vi "FindFocus.vi"(8 "error in (no error)":errorcluster, 11 "Transport":refnum<class "Transport.lvclass">) -> (0 "error out":errorcluster, 3 "Transport.lvclass":refnum<class "Transport.lvclass">)   [LabVIEW 2019, in "Transport.lvclass"]
uses:
  <userlib>/LevyLab/Transport/Transport/Transport.lvclass
  <userlib>/LevyLab/Instrument Framework/Instrument Types/Cryostat/Instrument.Cryostat.lvclass
  <userlib>/LevyLab/Transport/Control Experiment/Control Experiment.lvclass
  <userlib>/LevyLab/Krohn Hite 7008/Instrument.KH7008.lvclass
  <userlib>/LevyLab/Lockin-Multichannel/Instrument.Lockin/Instrument.Lockin.lvclass
  <userlib>/LevyLab/Transport/Control Experiment/Typedefs/Instruments--cluster.ctl
  <userlib>/LevyLab/Instrument Framework/Instrument Types/VSource/Instrument.VSource.lvclass
  <userlib>/LevyLab/Instrument Framework/Instrument Types/VNA/Instrument.VNA.lvclass
  <userlib>/LevyLab/Instrument Framework/Instrument Types/Strain/Instrument.Strain.lvclass
  <userlib>/LevyLab/Instrument Framework/Instrument Types/CBridge/Instrument.CBridge.lvclass
  <userlib>/LevyLab/Instrument Framework/Instrument Types/Delay Line/Instrument.DelayLine.lvclass
  <userlib>/LevyLab/Lockin-Multichannel/Instrument.Lockin/Typedefs/Results Type--Enum.ctl
panel:
  in  "set \"Vsg\" to initial value?":bool
  in  "Tab Control":enum32{"LockIn Control", "Data", "Other"}(tab)
  out "elapsed time (s)":u32=1660
  in  "Input":i32[](array[numeric])=[21]
  in  "End (um)":dbl=10.0 format="%#_3p"
  in  "Start (um)":dbl format="%#_3p"
  in  "Step (um)":dbl=0.1 format="%#_3p"
  in  "Experiment Comments":string
  in  "Experiment Folder":string="Focus Optimization xxxxxxxx"
  out "T (mK)":dbl=0.001
  in  "wait after setting Control (ms)":u32=2000
  in  "Initial wait (ms)":u32=1000
  in  "Sweep":enum16{"Vsg", "Vbg", "Z-height", ""}(ring)=enum."Z-height"
  in  "cycles (1,2,...)":i32=1 min=1 step=1
  in  "phase":dbl
  out "Field (T)":dbl=-0.0003 format="%#_13g"
  in  "function (ramp)":enum16{"Ramp", "Triangle", "Sine"}(ring)
  out "time b/w points (ms)":u32=2066
  in  "stop":bool
  out "Mean vs. Parameter":cluster{dbl[], dbl[]}[](graph)
  out "X Lockins":cluster{dbl[], dbl[]}[](graph)
  out "Y Lockins":cluster{dbl[], dbl[]}[](graph)
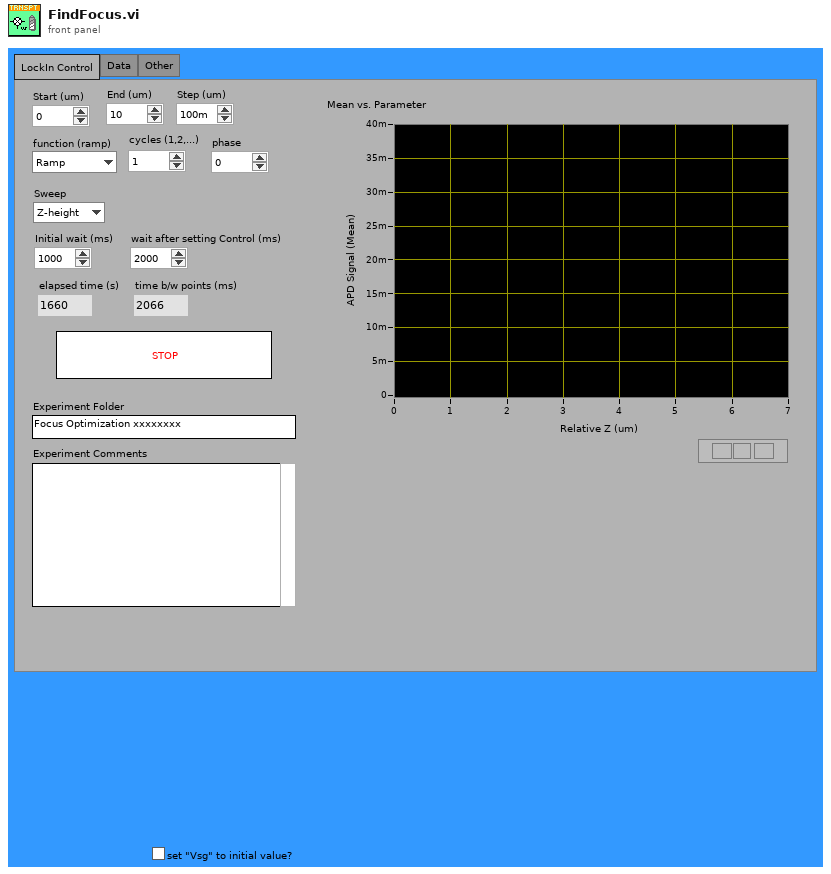
[diagram p1: front panel]
types:
  T1 = enum32{"Invalid", "Standard", "Closed", "Hidden", "Minimized", "Maximized"}
  T2 = enum32{"invalid app kind", "Development System", "Run Time System", "Student Edition", "Embedded LabVIEW", "Evaluation", "Custom"}
  T3 = typedef "Instrument.Lockin.lvclass/Results Type--Enum.ctl" = enum16{"X", "Y", "R", "Theta", "Mean"}
  T4 = typedef "Control Experiment.lvclass/Instruments--cluster.ctl" = cluster{"KH7008":refnum<class "Instrument.KH7008.lvclass">[], "Lockin":refnum<class "Instrument.Lockin.lvclass">, "Temperature":refnum<class "Instrument.Cryostat.lvclass">, "Magnet":refnum<class "Instrument.Cryostat.lvclass">, "Rotator":refnum<class "Instrument.Cryostat.lvclass">, "Level":refnum<class "Instrument.Cryostat.lvclass">, "Capacitance Bridge":refnum<class "Instrument.CBridge.lvclass">, "Delay Line":refnum<class "Instrument.DelayLine.lvclass">, "Strain Cell":refnum<class "Instrument.Strain.lvclass">, "VNA":refnum<class "Instrument.VNA.lvclass">, "Voltage Source":refnum<class "Instrument.VSource.lvclass">}
  T5 = cluster{"Core":cluster{"Current VI Reference":refnum<vi>, "Close Panel on Exit?":bool}, "Transport":refnum<class "Transport.lvclass">, "C.E.":refnum<class "Control Experiment.lvclass">, "Instruments":T4, "Sweep Values":dbl[], "Results (Dictionary)":cluster{"key":string, "value":dbl}[], "size":i32, "index":i32, "ms [0]":u32, "ms [i]":u32, "Execution:State":enum32{"Bad", "Idle", "Run top level", "Running"}}
  T6 = enum32{"Bad", "Idle", "Run top level", "Running"}
  T7 = cluster{"Current VI Reference":refnum<vi>, "Close Panel on Exit?":bool}
  T8 = cluster{"I-":i32, "I+":i32, "V1-":i32, "V1+":i32, "I2-":i32, "I2+":i32, "V2-":i32, "V2+":i32}
  T9 = typedef "Instrument.DAQ.lvclass/AO.Channel--Cluster--Array.ctl" = T10[]
  T10 = typedef "Instrument.DAQ.lvclass/AO.Channel--Cluster.ctl" = cluster{"Enable?":bool, "Channel":i32, "Amplitude":dbl, "Offset":dbl, "Frequency":dbl, "Phase":dbl, "Function":T11, "Sweeping?":bool}
  T11 = typedef "Instrument.DAQ.lvclass/AO.Channel.Function--Enum.ctl" = enum16{"Sine", "Triangle", "Square"}
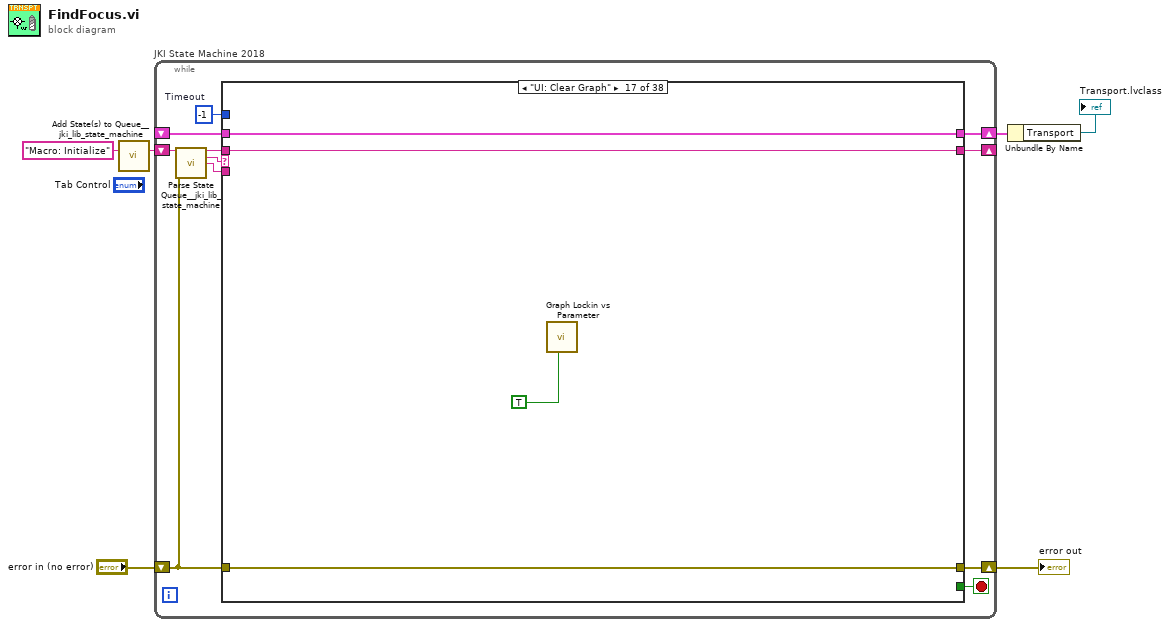
[diagram p0: block diagram]
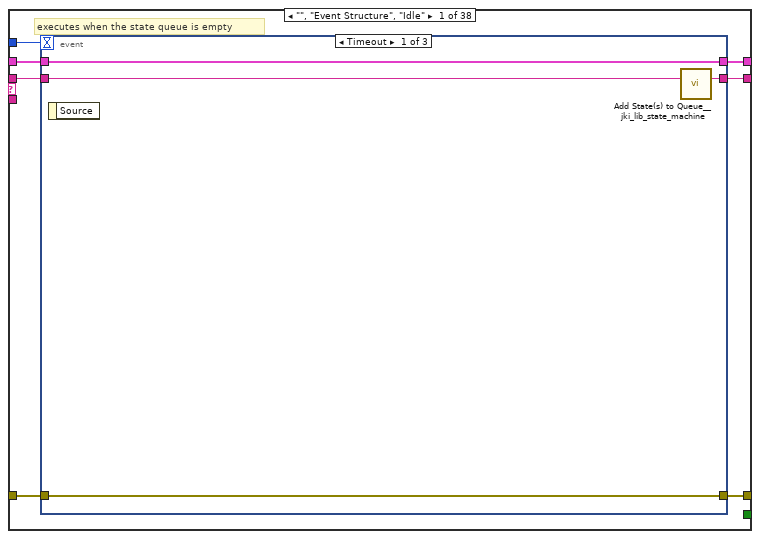
[diagram p2: hidden frame]
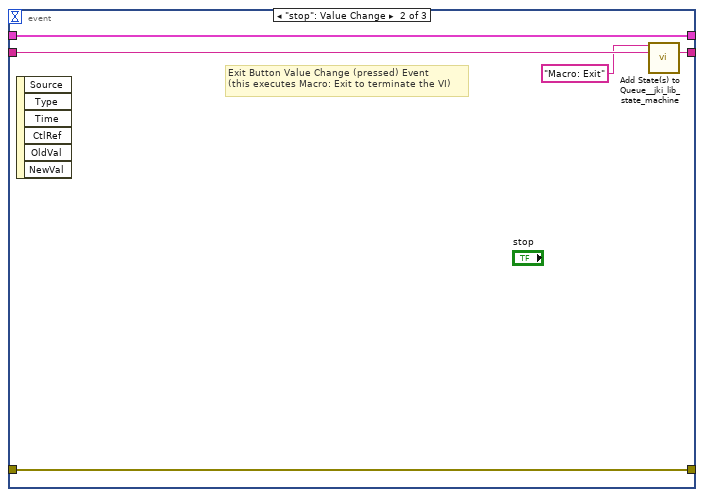
[diagram p3: hidden frame]
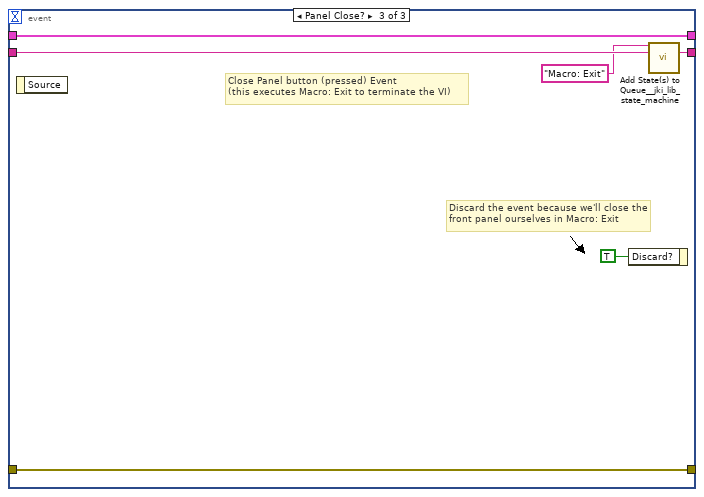
[diagram p4: hidden frame]
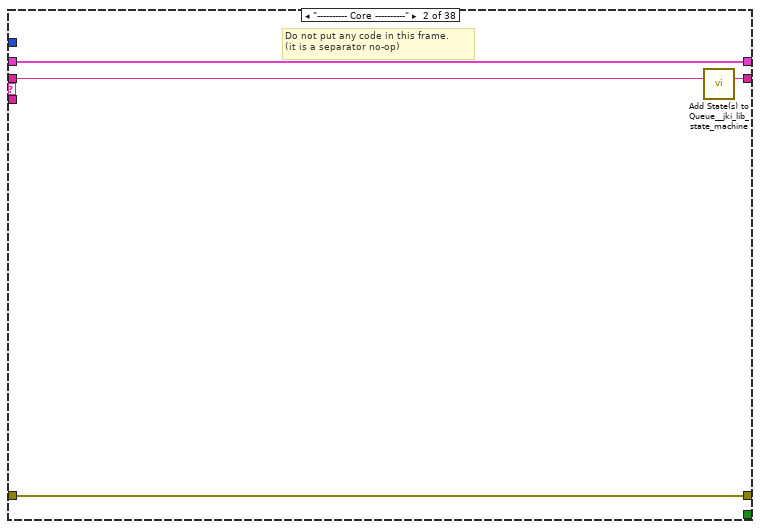
[diagram p5: hidden frame]
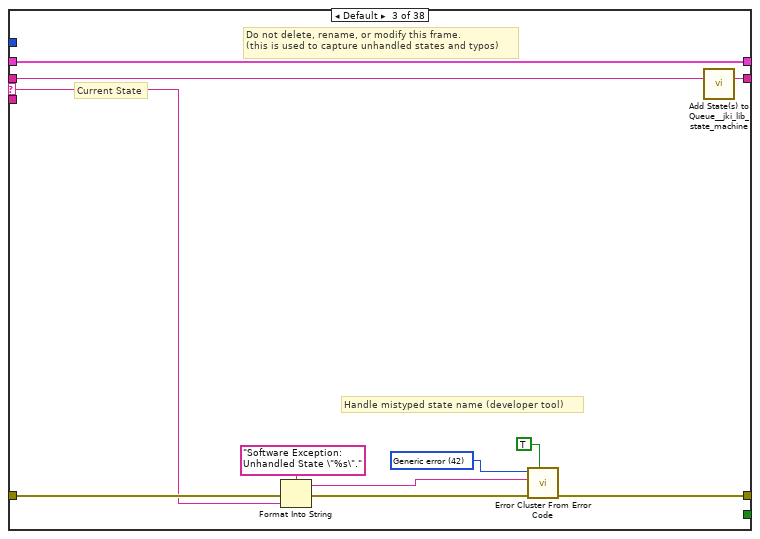
[diagram p6: hidden frame]
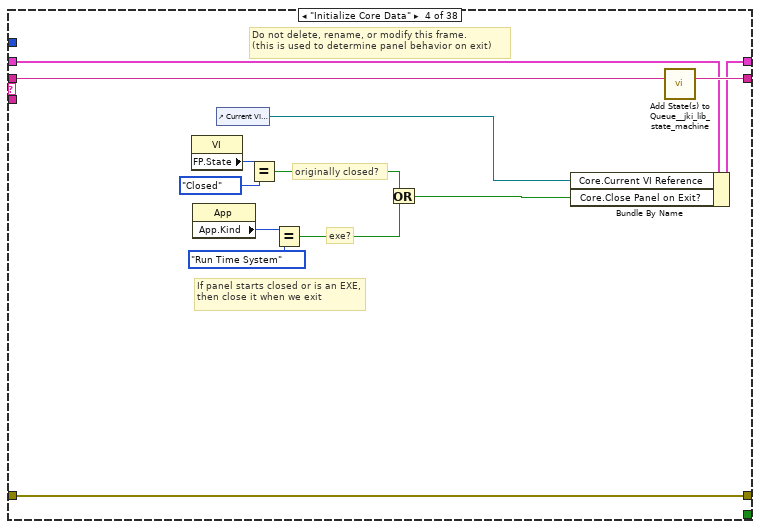
[diagram p7: hidden frame]
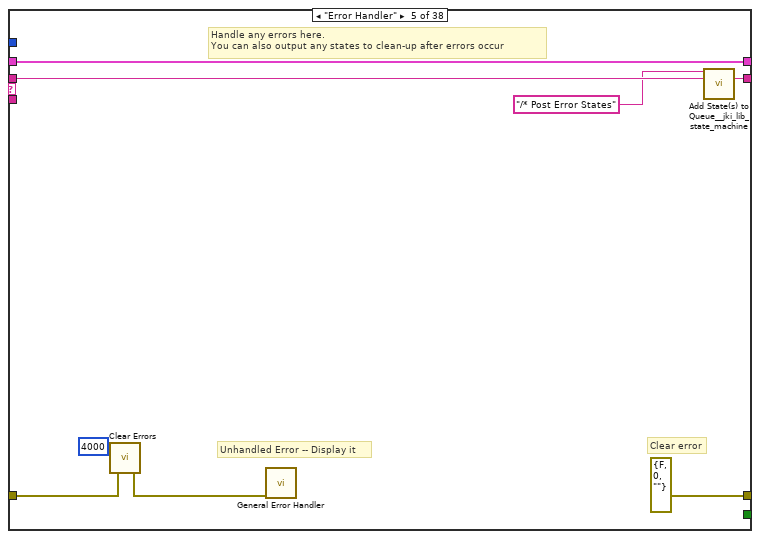
[diagram p8: hidden frame]
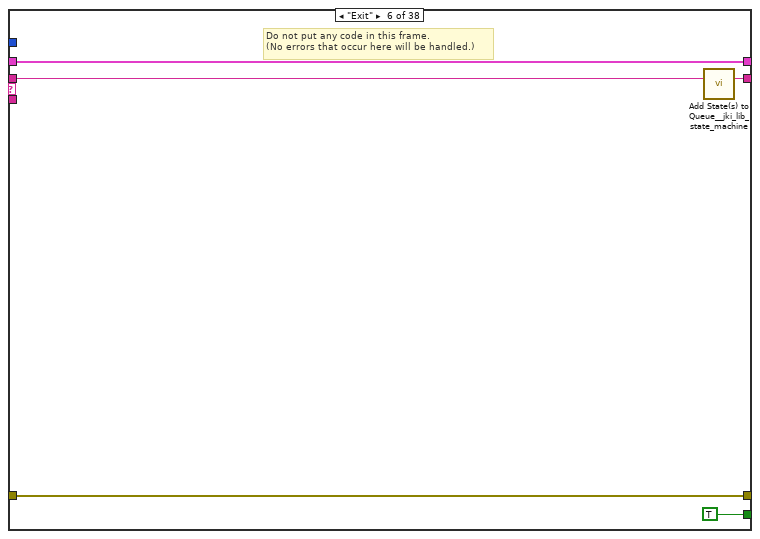
[diagram p9: hidden frame]
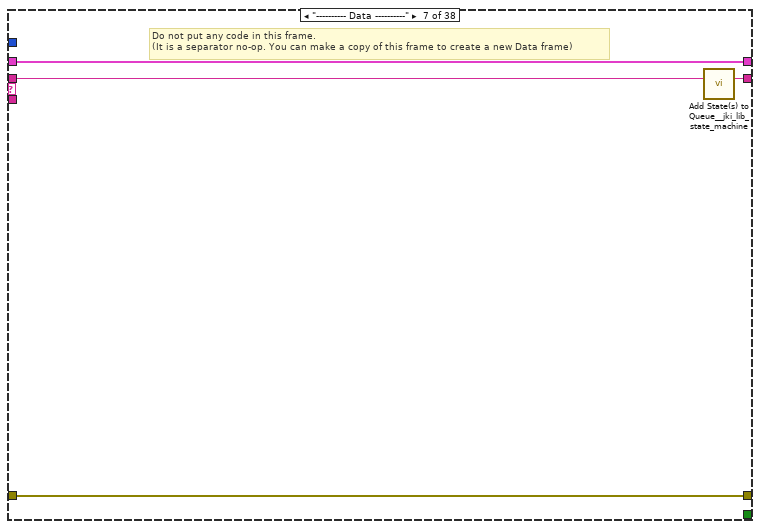
[diagram p10: hidden frame]
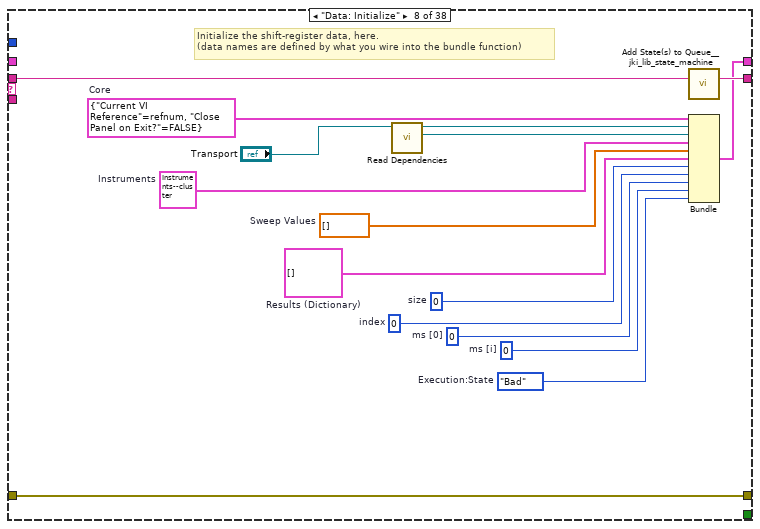
[diagram p11: hidden frame]
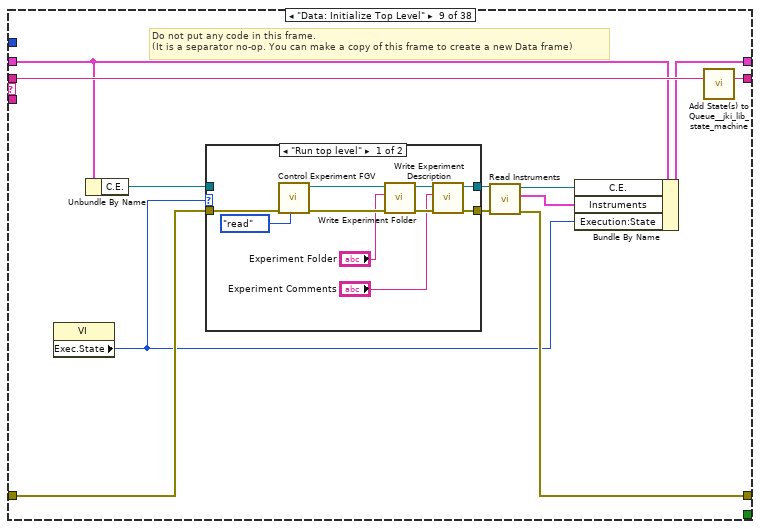
[diagram p12: hidden frame]
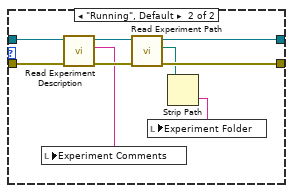
[diagram p13: hidden frame]
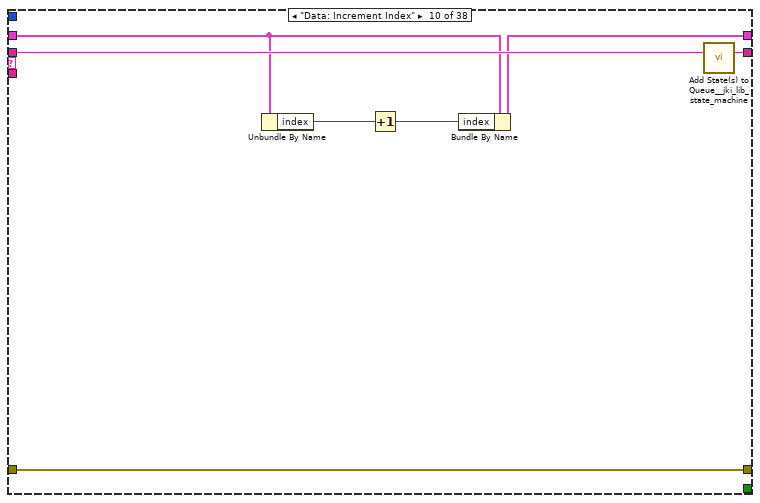
[diagram p14: hidden frame]
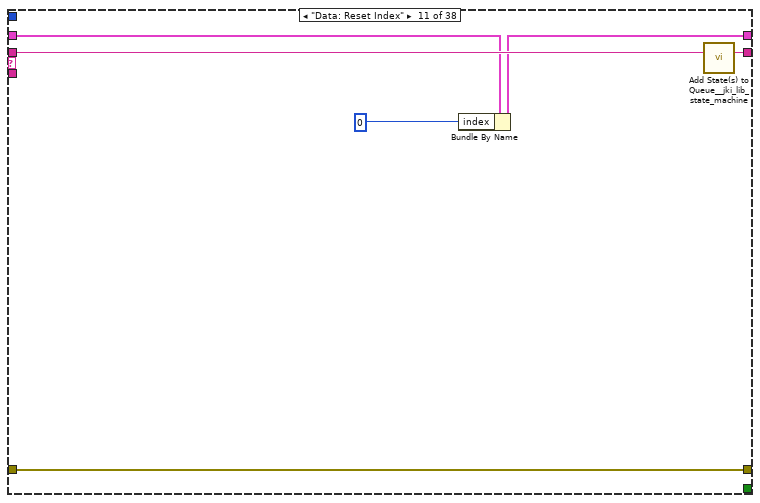
[diagram p15: hidden frame]
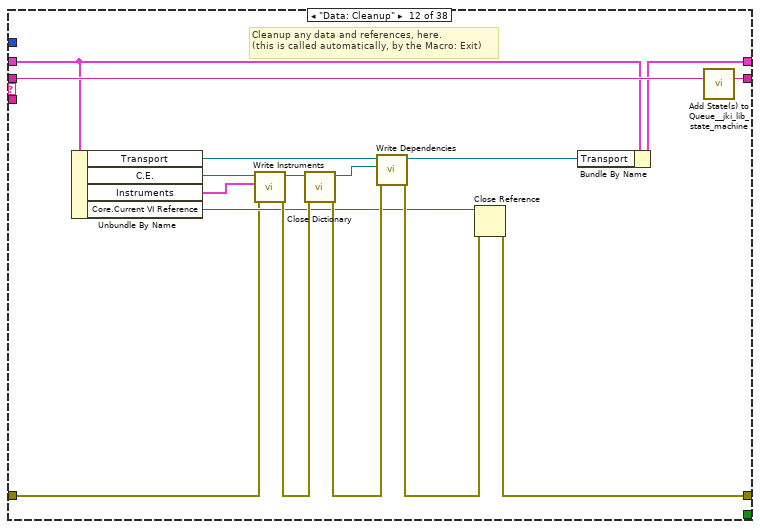
[diagram p16: hidden frame]
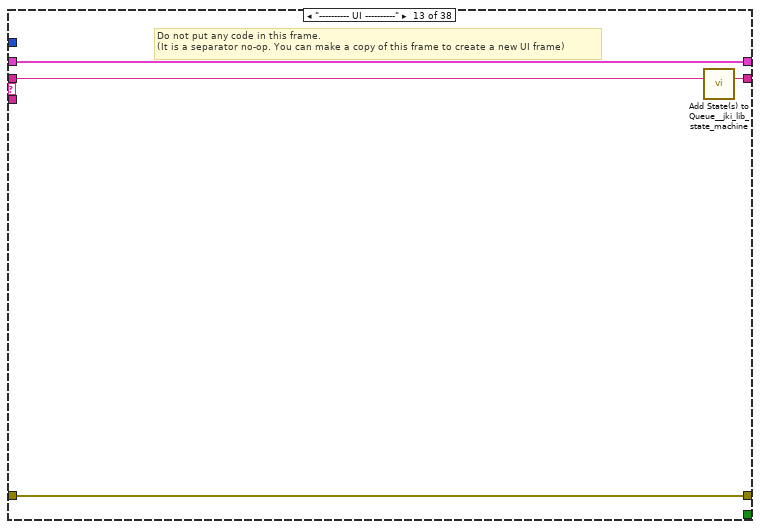
[diagram p17: hidden frame]
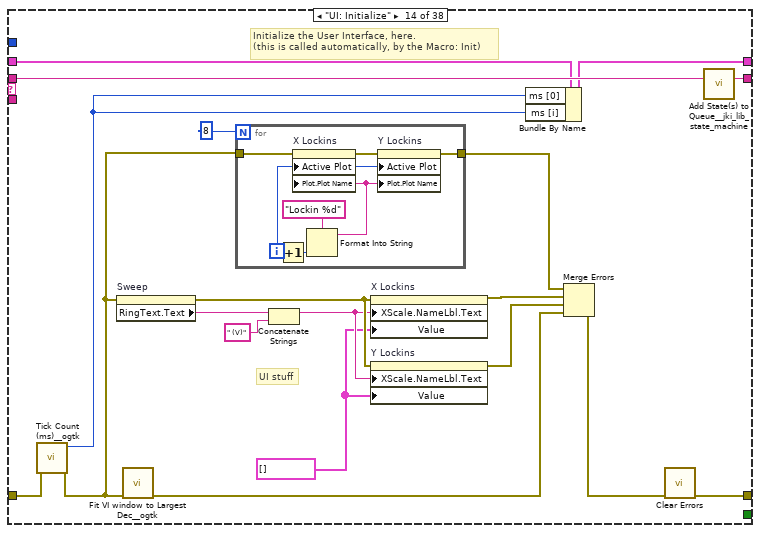
[diagram p18: hidden frame]
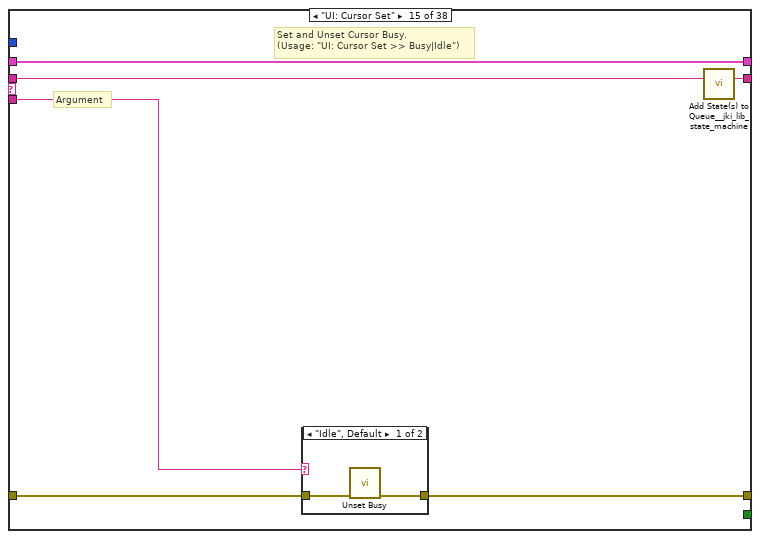
[diagram p19: hidden frame]
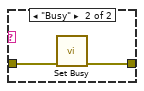
[diagram p20: hidden frame]
diagram:
  n1 = call <vilib>:"Add State(s) to Queue__jki_lib_state_machine.vi"("State(s) in (\"\")"="Macro: Initialize") -> ("States Out"=w6:string)  [unwired: 14 in]
  n2 = while "JKI State Machine 2018" {
    shift-right: [w10] -> w4
    shift-left: _ -> [w9]
    shift-right: [w13] -> w2
    shift-left: "error in (no error)" -> [w7]
    shift-right: [w12] -> _
    shift-left: w6 -> [w14]
    stop <- w11 stop-if-true
    w8 = -1  # Timeout
    n3 = call <vilib>:"Parse State Queue__jki_lib_state_machine.vi"("State Queue"=w14, "Error In (no error)"=w7) -> ("Remaining States"=w16:string, "Current State"=w17:string, "Arguments"=w15:string)  [unwired: 11 in]
    n4 = case shown="\"UI: Clear Graph\"" w17 {
      selector: w17 -> [_ _ w44 _ _ _ _ _ _ _ _ _ _ _ _ _ _ _ _ _ _ _ _ _ _ _ _ _ _ _ _ _ _ _ _ _ _ _]
      tunnel: w16 -> [w24 w43 w48 w67 w75 w80 w84 w100 w112 w138 w144 w160 w164 w183 w196 w216 w219 w233 w240 w309 w314 w336 w346 w350 w378 w390 w397 w411 w466 w479 w492 w505 w523 w555 w566 w570 w574 w583]
      tunnel: w15 -> [_ _ _ _ _ _ _ _ _ _ _ _ _ _ w191 _ _ _ w234 _ _ _ _ _ _ _ _ _ _ _ _ _ _ _ _ _ _ _]
      tunnel: w9 -> [w22 w40 w46 w60 w72 w78 w81 _ w103 w132 w141 w148 w161 w168 w194 w209 w220 w228 w236 w306 w312 w329 w343 w347 w366 w387 w393 w401 w463 w475 w489 w500 w518 w552 w562 w567 w571 w577]
      tunnel: [w21 w41 w50 w64 errorcluster {"status"=FALSE, "code"=0, "source"=""} ("error out") w77 w82 w97 w104 w136 w142 w145 w162 w173 w192 w214 w218 w222 w237 w307 w310 w334 w344 w348 w356 w388 w394 w405 w464 w471 w483 w496 w514 w546 w557 w568 w572 w580] -> w13
      tunnel: w7 -> [w20 w41 w49 w64 w69 w77 w82 w97 w105 w136 w142 w146 w162 w170 w193 w214 w218 w230 w238 w307 w310 w334 w344 w348 w363 w388 w395 w404 w464 w476 w487 w497 w521 w547 w558 w568 w572 w579]
      tunnel: [w23 w42 w47 w66 w74 w79 w83 w99 w111 w137 w143 w159 w163 w182 w195 w215 w219 w232 w239 w308 w313 w335 w345 w349 w377 w389 w396 w410 w465 w478 w491 w504 w522 w554 w565 w569 w573 w582] -> w12
      tunnel: [_ _ _ _ _ TRUE _ _ _ _ _ _ _ _ _ _ _ _ _ _ _ _ _ _ _ _ _ _ _ _ _ _ _ _ _ _ _ _] -> w11
      tunnel: [w19 w40 w46 w65 w72 w78 w81 w98 w102 w135 w140 w147 w161 w167 w194 w209 w220 w227 w236 w306 w312 w329 w343 w347 w369 w387 w393 w402 w463 w474 w488 w499 w519 w553 w563 w567 w571 w576] -> w10
      tunnel: w8 -> [w18 _ _ _ _ _ _ _ _ _ _ _ _ _ _ _ _ _ _ _ _ _ _ _ _ _ _ _ _ _ _ _ _ _ _ _ _ _]
      frame "", "Event Structure", "Idle" {
        # "executes when the state queue is empty"
        n5 = event shown="[0] Timeout" {
          selector: _ -> [_ _ _]
          dyn-events: _ -> [_ _ _]
          timeout: w18 -> [_ _ _]
          tunnel: w24 -> [w28 w33 w39]
          tunnel: [w27 w32 w38] -> w23
          tunnel: w22 -> [w25 w30 w36]
          tunnel: [w26 w31 w37] -> w21
          tunnel: w20 -> [w26 w31 w37]
          tunnel: [w25 w30 w36] -> w19
          event Timeout {
            n6 = event-data() -> ()  [unwired: 1 in, 1 out]
            n7 = call <vilib>:"Add State(s) to Queue__jki_lib_state_machine.vi"("State(s) in (\"\")"=w28) -> ("States Out"=w27:string)  [unwired: 14 in]
          }
          event "stop": Value Change {
            # "Exit Button Value Change (pressed) Event\n(this executes Macro: Exit to terminate the VI)"
            n8 = event-data() -> ()  [unwired: 1 in, 6 out]
            n9 = call <vilib>:"Add State(s) to Queue__jki_lib_state_machine.vi"("State(s) in Front (\"\")"="Macro: Exit", "State(s) in (\"\")"=w33) -> ("States Out"=w32:string)  [unwired: 13 in]
          }
          event Panel Close? {
            # "Discard the event because we'll close the front panel ourselves in Macro: Exit"
            # "Close Panel button (pressed) Event\n(this executes Macro: Exit to terminate the VI)"
            n10 = event-data() -> ()  [unwired: 1 in, 1 out]
            n11 = event-data("Discard?"=TRUE) -> ()  [unwired: 1 in, 1 out]
            n12 = call <vilib>:"Add State(s) to Queue__jki_lib_state_machine.vi"("State(s) in Front (\"\")"="Macro: Exit", "State(s) in (\"\")"=w39) -> ("States Out"=w38:string)  [unwired: 13 in]
          }
        }
      }
      frame "---------- Core ----------" {
        # "Do not put any code in this frame.\n(it is a separator no-op)"
        n13 = call <vilib>:"Add State(s) to Queue__jki_lib_state_machine.vi"("State(s) in (\"\")"=w43) -> ("States Out"=w42:string)  [unwired: 14 in]
      }
      frame Default {
        w53 = 42 items=["No error", "Argument error", "Memory is full", "Out of zone", "End of file", "File already open", "Generic file I/O error", "File not found", "File permission error", "Disk is full", "Duplicate path", "Too many files open", "System feature not enabled", "Resource file not found", "Cannot add resource", "Resource not found", "Image not found", "Image memory error", "Pen does not exist", "Config type invalid", "Config token not found", "Config parse error", "Config memory error", "Bad external code format", "Bad external code offset", "External code not present", "Null window", "Destroy window error", "Null menu", "Print aborted", "Bad print record", "Print driver error", "Windows error during printing", "Memory error during printing", "Print dialog error", "Generic print error", "Invalid device refnum", "Device not found", "Device parameter error", "Device unit error", "Cannot open device", "Device call aborted", "Generic error", "Cancelled by user", "Object ID too low", "Object ID too high", "Object not in heap", "Unknown heap", "Unknown object (invalid DefProc)", "Unknown object (DefProc not in table)", "Message out of range", "Invalid (null) method", "Unknown message", "Manager call not supported", "Bad address", "Network operation in progress", "Network operation timed out", "Connection is busy", "Network attribute not supported", "Network error", "Address in use", "System out of memory", "Connection aborted", "Connection refused", "Not connected", "Already connected", "Connection closed", "Initialization error (interapplication manager)", "Bad occurrence", "Wait on unbound occurrence handler", "Occurrence queue overflow", "Datalog type conflict", "Unused", "Unrecognized type (interapplication manager)", "Memory corrupt", "Failed to make temporary DLL", "Old CIN version", "Drag socket not found", "Failed to load drop-object", "Failed to register OLE object", "Failed to release OLE object", "Format specifier type mismatch", "Unknown format specifier", "Too few format specifiers", "Too many format specifiers", "Scan failed", "Newer CIN version", "Error converting to variant", "Runtime menu error", "Password tampered", "Variant attribute not found", "Incompatible variant data type", "Event data is not available", "Event Store is not present", "Occurrence is not found", "Event Queue is not created", "Event info is not available", "Refnum passed is NULL", "Error retrieving Class GUID", "Error retrieving CoClass GUID", "Error retrieving TypeLib GUID.", "Bad built application magic bytes.", "Specific driver is different from the specific driver associated with the Logical Name.", "There is no session opened to the class driver.", "Max Error", "MAX - Error with config objects", "MAX - Error loading configuration", "MAX - Group not supported"]
        # "Current State"
        # "Do not delete, rename, or modify this frame.\n(this is used to capture unhandled states and typos)"
        # "Handle mistyped state name (developer tool)"
        n14 = Format Into String(format string="Software Exception: Unhandled State \"%s\"." ("message"), error in=w49, w44) -> (resulting string=w52:string, error out=w51:errorcluster)  [unwired: 1 in]
        n15 = call <vilib>:"Error Cluster From Error Code.vi"("show call chain? (False)"=TRUE, "error in (no error)"=w51, "error message (\"\")"=w52, "error code (0)"=w53) -> ("error out"=w50:errorcluster)  [unwired: 5 in]
        n16 = call <vilib>:"Add State(s) to Queue__jki_lib_state_machine.vi"("State(s) in (\"\")"=w48) -> ("States Out"=w47:string)  [unwired: 14 in]
      }
      frame "Initialize Core Data" {
        # "Do not delete, rename, or modify this frame.\n(this is used to determine panel behavior on exit)"
        # "originally closed?"
        # "exe?"
        # "If panel starts closed or is an EXE, then close it when we exit"
        n17 = property class="VI"() -> ("FP.State"=w57:T1)  [unwired: 2 in, 2 out]
        n18 = property class="App"() -> ("App.Kind"=w63:T2)  [unwired: 2 in, 2 out]
        n19 = control-ref of="Current VI Reference"() -> (w58:refnum<vi>)
        n20 = Equal?(x=w57, y=T1."Closed" ("Front Panel Window:State")) -> (x = y?=w55:bool)
        n21 = Equal?(x=w63, y=T2."Run Time System" ("Application:Kind")) -> (x = y?=w61:bool)
        n22 = Or(x=w55, y=w61) -> (x .or. y?=w59:bool)
        n23 = Bundle By Name(cluster=w60, "Core.Current VI Reference"=w58, "Core.Close Panel on Exit?"=w59) -> (w65:T5)
        n24 = call <vilib>:"Add State(s) to Queue__jki_lib_state_machine.vi"("State(s) in (\"\")"=w67) -> ("States Out"=w66:string)  [unwired: 14 in]
      }
      frame "Error Handler" {
        # "Unhandled Error -- Display it"
        # "Handle any errors here.\nYou can also output any states to clean-up after errors occur"
        # "Clear error"
        n25 = call <vilib>:"Clear Errors.vi"("error in (no error)"=w69, "specific error code to clear (0: all)"=4000) -> ("error out"=w68:errorcluster)  [unwired: 4 in, 1 out]
        n26 = call <vilib>:"General Error Handler.vi"("error in (no error)"=w68) -> ()  [unwired: 10 in, 5 out]
        n27 = call <vilib>:"Add State(s) to Queue__jki_lib_state_machine.vi"("State(s) in Front (\"\")"="/* Post Error States", "State(s) in (\"\")"=w75) -> ("States Out"=w74:string)  [unwired: 13 in]
      }
      frame "Exit" {
        # "Do not put any code in this frame.\n(No errors that occur here will be handled.)"
        n28 = call <vilib>:"Add State(s) to Queue__jki_lib_state_machine.vi"("State(s) in (\"\")"=w80) -> ("States Out"=w79:string)  [unwired: 14 in]
      }
      frame "---------- Data ----------" {
        # "Do not put any code in this frame.\n(It is a separator no-op. You can make a copy of this frame to create a new Data frame)"
        n29 = call <vilib>:"Add State(s) to Queue__jki_lib_state_machine.vi"("State(s) in (\"\")"=w84) -> ("States Out"=w83:string)  [unwired: 14 in]
      }
      frame "Data: Initialize" {
        w85 = cluster{"key":string, "value":dbl}[] []  # Results (Dictionary)
        w89 = T6."Bad"  # Execution:State
        w90 = 0  # size
        w91 = u32 0  # ms [i]
        w92 = u32 0  # ms [0]
        w93 = 0  # index
        w94 = dbl[] []  # Sweep Values
        w95 = T4 {"KH7008"=[], "Lockin"=refnum, "Temperature"=refnum, "Magnet"=refnum, "Rotator"=refnum, "Level"=refnum, "Capacitance Bridge"=refnum, "Delay Line"=refnum, "Strain Cell"=refnum, "VNA"=refnum, "Voltage Source"=refnum}  # Instruments
        w96 = T7 {"Current VI Reference"=refnum, "Close Panel on Exit?"=FALSE}  # Core
        # "Initialize the shift-register data, here.\n(data names are defined by what you wire into the bundle function)"
        n30 = call <userlib>:"Read Dependencies.vi"("Transport"="Transport") -> ("C.E."=w87:refnum<class "Control Experiment.lvclass">, "Transport"=w86:refnum<class "Transport.lvclass">)  [unwired: 8 in, 1 out]
        n31 = call <vilib>:"Add State(s) to Queue__jki_lib_state_machine.vi"("State(s) in (\"\")"=w100) -> ("States Out"=w99:string)  [unwired: 14 in]
        n32 = Bundle("Core"=w96, "Transport"=w86, "C.E."=w87, "Instruments"=w95, "Sweep Values"=w94, "Results (Dictionary)"=w85, "size"=w90, "index"=w93, "ms [0]"=w92, "ms [i]"=w91, "Execution:State"=w89) -> (w98:T5)  [unwired: 1 in]
      }
      frame "Data: Initialize Top Level" {
        # "Do not put any code in this frame.\n(It is a separator no-op. You can make a copy of this frame to create a new Data frame)"
        n33 = property class="VI"() -> ("Exec.State"=w101:T6)  [unwired: 2 in, 2 out]
        n34 = Unbundle By Name(w103) -> ("C.E."=w106:refnum<class "Control Experiment.lvclass">)
        n35 = case shown="\"Run top level\"" w101 {
          tunnel: w105 -> [w122 w130]
          tunnel: [w117 w126] -> w107
          tunnel: [w116 w127] -> w108
          tunnel: w106 -> [_ w131]
          frame "Run top level" {
            n36 = call <userlib>:"Control Experiment FGV.vi"("Function"=enum16{"read", "write"}."read", "error in (no error)"=w122) -> ("error out"=w120:errorcluster, "Control Experiment.lvclass out"=w121:refnum<class "Control Experiment.lvclass">)  [unwired: 8 in]
            n37 = call <userlib>:"Write Experiment Folder.vi"("error in (no error)"=w120, "Experiment Folder"="Experiment Folder", "Control Experiment in"=w121) -> ("error out"=w118:errorcluster, "Control Experiment out"=w119:refnum<class "Control Experiment.lvclass">)  [unwired: 7 in]
            n38 = call <userlib>:"Write Experiment Description.vi"("error in (no error)"=w118, "Experiment Description"="Experiment Comments", "Control Experiment in"=w119) -> ("error out"=w117:errorcluster, "Control Experiment out"=w116:refnum<class "Control Experiment.lvclass">)  [unwired: 7 in]
          }
          frame "Running", Default {
            n39 = call <userlib>:"Read Experiment Description.vi"("error in (no error)"=w130, "Control Experiment in"=w131) -> ("error out"=w129:errorcluster, "Experiment Description"=w124:string, "Control Experiment out"=w128:refnum<class "Control Experiment.lvclass">)  [unwired: 7 in]
            n40 = local write "Experiment Comments"(w124) -> ()
            n41 = call <userlib>:"Read Experiment Path.vi"("error in (no error)"=w129, "Control Experiment in"=w128) -> ("error out"=w126:errorcluster, "Experiment Path"=w125:path, "Control Experiment out"=w127:refnum<class "Control Experiment.lvclass">)  [unwired: 7 in]
            n42 = Strip Path(path=w125) -> (name=w123:string)  [unwired: 1 out]
            n43 = local write "Experiment Folder"(w123) -> ()
          }
        }
        n44 = call <userlib>:"Read Instruments.vi"("error in (no error)"=w107, "Control Experiment in"=w108) -> ("error out"=w104:errorcluster, "Instruments"=w110:T4, "Control Experiment out"=w109:refnum<class "Control Experiment.lvclass">)  [unwired: 7 in]
        n45 = Bundle By Name(cluster=w103, "C.E."=w109, "Instruments"=w110, "Execution:State"=w101) -> (w102:T5)
        n46 = call <vilib>:"Add State(s) to Queue__jki_lib_state_machine.vi"("State(s) in (\"\")"=w112) -> ("States Out"=w111:string)  [unwired: 14 in]
      }
      frame "Data: Increment Index" {
        n47 = Unbundle By Name(w132) -> ("index"=w134:i32)
        n48 = Increment(x=w134) -> (x+1=w133:i32)
        n49 = Bundle By Name(cluster=w132, "index"=w133) -> (w135:T5)
        n50 = call <vilib>:"Add State(s) to Queue__jki_lib_state_machine.vi"("State(s) in (\"\")"=w138) -> ("States Out"=w137:string)  [unwired: 14 in]
      }
      frame "Data: Reset Index" {
        n51 = Bundle By Name(cluster=w141, "index"=0) -> (w140:T5)
        n52 = call <vilib>:"Add State(s) to Queue__jki_lib_state_machine.vi"("State(s) in (\"\")"=w144) -> ("States Out"=w143:string)  [unwired: 14 in]
      }
      frame "Data: Cleanup" {
        # "Cleanup any data and references, here.\n(this is called automatically, by the Macro: Exit)"
        n53 = Unbundle By Name(w148) -> ("Transport"=w157:refnum<class "Transport.lvclass">, "C.E."=w155:refnum<class "Control Experiment.lvclass">, "Instruments"=w153:T4, "Core.Current VI Reference"=w149:refnum<vi>)
        n54 = call <userlib>:"Write Instruments.vi"("error in (no error)"=w146, "Instruments"=w153, "Control Experiment in"=w155) -> ("error out"=w152:errorcluster, "Control Experiment out"=w154:refnum<class "Control Experiment.lvclass">)  [unwired: 7 in]
        n55 = call <userlib>:"Close Dictionary.vi"("error in (no error)"=w152, "Control Experiment in"=w154) -> ("error out"=w151:errorcluster, "Control Experiment out"=w156:refnum<class "Control Experiment.lvclass">)  [unwired: 8 in]
        n56 = call <userlib>:"Write Dependencies.vi"("error in (no error)"=w151, "Control Experiment"=w156, "Transport in"=w157) -> ("error out"=w150:errorcluster, "Transport out"=w158:refnum<class "Transport.lvclass">)  [unwired: 7 in]
        n57 = Close Reference(reference=w149, error in (no error)=w150) -> (error out=w145:errorcluster)
        n58 = Bundle By Name(cluster=w148, "Transport"=w158) -> (w147:T5)
        n59 = call <vilib>:"Add State(s) to Queue__jki_lib_state_machine.vi"("State(s) in (\"\")"=w160) -> ("States Out"=w159:string)  [unwired: 14 in]
      }
      frame "---------- UI ----------" {
        # "Do not put any code in this frame.\n(It is a separator no-op. You can make a copy of this frame to create a new UI frame)"
        n60 = call <vilib>:"Add State(s) to Queue__jki_lib_state_machine.vi"("State(s) in (\"\")"=w164) -> ("States Out"=w163:string)  [unwired: 14 in]
      }
      frame "UI: Initialize" {
        w165 = cluster{dbl[], dbl[]}[] [] ("G4T")
        # "UI stuff"
        # "Initialize the User Interface, here.\n(this is called automatically, by the Macro: Init)"
        n61 = call <userlib>:"Tick Count (ms)__ogtk.vi"("error in (no error)"=w170) -> ("error out"=w169:errorcluster, "millisecond timer value"=w166:u32)  [unwired: 9 in]
        n62 = property on="Sweep" class="Enum (strict)"(error in=w169) -> (error out=w178:errorcluster, "RingText.Text"=w176:string)  [unwired: 1 in, 1 out]
        n63 = call <userlib>:"Fit VI window to Largest Dec__ogtk.vi"("error in (no error)"=w169) -> ("error out"=w172:errorcluster)  [unwired: 5 in, 1 out]
        n64 = for {
          N: 8 -> [_]
          tunnel: [w184] -> w179
          tunnel: w169 -> [w189]
          i -> [w187]
          n65 = Increment(x=w187) -> (x+1=w185:i32)
          n66 = Format Into String(format string="Lockin %d", w185) -> (resulting string=w188:string)  [unwired: 2 in, 1 out]
          n67 = property on="X Lockins" class="XYGraph (strict)"(error in=w189, "Active Plot"=w187, "Plot.Plot Name"=w188) -> (error out=w186:errorcluster)  [unwired: 1 in, 1 out]
          n68 = property on="Y Lockins" class="XYGraph (strict)"(error in=w186, "Active Plot"=w187, "Plot.Plot Name"=w188) -> (error out=w184:errorcluster)  [unwired: 1 in, 1 out]
        }
        n69 = Concatenate Strings(w176, " (V)" ("string")) -> (w177:string)
        n70 = property on="X Lockins" class="XYGraph (strict)"(error in=w178, "XScale.NameLbl.Text"=w177, "Value"=w165) -> (error out=w180:errorcluster)  [unwired: 1 in, 1 out]
        n71 = property on="Y Lockins" class="XYGraph (strict)"(error in=w178, "XScale.NameLbl.Text"=w177, "Value"=w165) -> (error out=w181:errorcluster)  [unwired: 1 in, 1 out]
        n72 = Bundle By Name(cluster=w168, "ms [0]"=w166, "ms [i]"=w166) -> (w167:T5)
        n73 = Merge Errors(w179, w180, w181, w172) -> (w171:errorcluster)
        n74 = call <vilib>:"Clear Errors.vi"("error in (no error)"=w171) -> ("error out"=w173:errorcluster)  [unwired: 5 in, 1 out]
        n75 = call <vilib>:"Add State(s) to Queue__jki_lib_state_machine.vi"("State(s) in (\"\")"=w183) -> ("States Out"=w182:string)  [unwired: 14 in]
      }
      frame "UI: Cursor Set" {
        # "Argument"
        # "Set and Unset Cursor Busy.\n(Usage: \"UI: Cursor Set >> Busy|Idle\")"
        n76 = case shown="\"Idle\", Default" w191 {
          tunnel: w193 -> [w198 w200]
          tunnel: [w197 w199] -> w192
          frame "Idle", Default {
            n77 = call <vilib>:"Unset Busy.vi"("error in (no error)"=w198) -> ("error out"=w197:errorcluster)  [unwired: 10 in]
          }
          frame "Busy" {
            n78 = call <vilib>:"Set Busy.vi"("error in (no error)"=w200) -> ("error out"=w199:errorcluster)  [unwired: 9 in, 1 out]
          }
        }
        n79 = call <vilib>:"Add State(s) to Queue__jki_lib_state_machine.vi"("State(s) in (\"\")"=w196) -> ("States Out"=w195:string)  [unwired: 14 in]
      }
      frame "UI: Update Graphs" {
        n80 = Unbundle By Name(w209) -> ("index"=w210:i32, "Sweep Values"=w211:dbl[], "C.E."=w213:refnum<class "Control Experiment.lvclass">, "Results (Dictionary)"=w208:cluster{"key":string, "value":dbl}[])
        n81 = call <userlib>:"Get Channel Indices.vi"("Control Experiment in"=w213) -> ("Indices"=w212:T8)  [unwired: 8 in, 2 out]
        n82 = call <userlib>:"Parse Results (all).vi"("Type"=Results_Type--Enum."Mean", "Results (Dictionary)"=w208) -> ("Data"=w202:dbl[])  [unwired: 6 in, 3 out]
        n83 = Unbundle By Name(w212) -> ()  [unwired: 3 out]
        n84 = call <userlib>:"Results (Dictionary) to X and Y Arrays.vi"("Results (Dictionary)"=w208) -> ("X"=w204:dbl[])  [unwired: 9 in, 1 out]
        n85 = Index Array(array=w211, index=w210) -> (element=w203:dbl)
        n86 = Equal To 0?(x=w210) -> ()  [unwired: 1 out]
        n87 = property on="Mean vs. Parameter" class="XYGraph (strict)"("XScale.Multiplier"=8.0 ("X Scale.Offset and Multiplier:Multiplier")) -> ()  [unwired: 2 in, 2 out]
        n88 = call <userlib>:"Graph Lockin vs Parameter.vi"("Parameter"=w203, "Y[ ]"=w202, "X[ ]"=w204) -> ("Y vs Parameter"=→"Y Lockins" →"Mean vs. Parameter":cluster{dbl[], dbl[]}[], "X vs Parameter"=→"X Lockins":cluster{dbl[], dbl[]}[])  [unwired: 7 in]
        n89 = call <vilib>:"Add State(s) to Queue__jki_lib_state_machine.vi"("State(s) in (\"\")"=w216) -> ("States Out"=w215:string)  [unwired: 14 in]
      }
      frame "UI: Clear Graph" {
        n90 = call <userlib>:"Graph Lockin vs Parameter.vi"("reset?"=TRUE ("Reset")) -> ()  [unwired: 9 in, 2 out]
      }
      frame "UI: Update Timer" {
        n91 = Unbundle By Name(w228) -> ("ms [0]"=w229:u32)
        n92 = call <userlib>:"Tick Count (ms)__ogtk.vi"("error in (no error)"=w230) -> ("error out"=w223:errorcluster, "millisecond timer value"=w221:u32)  [unwired: 9 in]
        n93 = Subtract(x=w221, y=w229) -> (x-y=w225:u32)
        n94 = call <userlib>:"MGI Milliseconds Since Last Call.vi"("Error In"=w223) -> ("ms"=→"time b/w points (ms)":u32, "Error Out"=w222:errorcluster)  [unwired: 5 in]
        n95 = Divide(x=w225, y=u32 1000 ("x")) -> (x/y=→"elapsed time (s)":dbl)
        n96 = Bundle By Name(cluster=w228, "ms [i]"=w221) -> (w227:T5)
        n97 = call <vilib>:"Add State(s) to Queue__jki_lib_state_machine.vi"("State(s) in (\"\")"=w233) -> ("States Out"=w232:string)  [unwired: 14 in]
      }
      frame "UI: Front Panel State" {
        # "Argument"
        # "Set Front Panel Open or Closed\n(Usage: \"UI: Front Panel State >> Open|Close\")"
        n98 = Unbundle By Name(w236) -> ("Core.Current VI Reference"=w235:refnum<vi>)
        n99 = case shown="\"Minimize\", \"Minimized\"" w234 {
          tunnel: w238 -> [w246 w261 w272 w285 w298]
          tunnel: [w248 w262 w274 w287 w300] -> w237
          tunnel: w235 -> [w247 w259 w273 w286 w299]
          frame "Open", "Standard", Default {
            w241 = T1."Standard" ("State")
            n100 = property class="VI"(reference=w247, error in=w246) -> (reference out=w244:refnum<vi>, error out=w245:errorcluster, "FP.State"=w243:T1)
            n101 = Not Equal?(x=w243, y=w241) -> (x != y?=w242:bool)
            n102 = case shown="True" w242 {
              tunnel: [w252 w254] -> w248
              tunnel: w245 -> [w251 w254]
              tunnel: w244 -> [w250 _]
              tunnel: w241 -> [w249 _]
              frame True {
                n103 = invoke class="VI" method="FP.Open"(reference=w250, error in=w251, "Activate"=TRUE, "State"=w249) -> (error out=w252:errorcluster)  [unwired: 1 in, 4 out]
              }
              frame False {
              }
            }
          }
          frame "Close", "Closed" {
            n104 = property class="VI"(reference=w259, error in=w261) -> (reference out=w258:refnum<vi>, error out=w260:errorcluster, "FP.State"=w256:T1)
            n105 = Not Equal?(x=w256, y=T1."Closed" ("Front Panel Window:State")) -> (x != y?=w255:bool)
            n106 = case shown="True" w255 {
              tunnel: [w263 w266] -> w262
              tunnel: w260 -> [w263 w265]
              tunnel: w258 -> [_ w264]
              frame False {
              }
              frame True {
                n107 = invoke class="VI" method="FP.Close"(reference=w264, error in=w265) -> (error out=w266:errorcluster)  [unwired: 1 in, 2 out]
              }
            }
          }
          frame "Hidden", "Hide" {
            w267 = T1."Hidden" ("State")
            n108 = property class="VI"(reference=w273, error in=w272) -> (reference out=w270:refnum<vi>, error out=w271:errorcluster, "FP.State"=w269:T1)
            n109 = Not Equal?(x=w269, y=w267) -> (x != y?=w268:bool)
            n110 = case shown="True" w268 {
              tunnel: [w278 w279] -> w274
              tunnel: w271 -> [w277 w279]
              tunnel: w270 -> [w276 _]
              tunnel: w267 -> [w275 _]
              frame True {
                n111 = invoke class="VI" method="FP.Open"(reference=w276, error in=w277, "State"=w275) -> (error out=w278:errorcluster)  [unwired: 2 in, 4 out]
              }
              frame False {
              }
            }
          }
          frame "Minimize", "Minimized" {
            w280 = T1."Minimized" ("State")
            n112 = property class="VI"(reference=w286, error in=w285) -> (reference out=w283:refnum<vi>, error out=w284:errorcluster, "FP.State"=w282:T1)
            n113 = Not Equal?(x=w282, y=w280) -> (x != y?=w281:bool)
            n114 = case shown="True" w281 {
              tunnel: [w291 w292] -> w287
              tunnel: w284 -> [w290 w292]
              tunnel: w283 -> [w289 _]
              tunnel: w280 -> [w288 _]
              frame True {
                n115 = invoke class="VI" method="FP.Open"(reference=w289, error in=w290, "State"=w288) -> (error out=w291:errorcluster)  [unwired: 2 in, 4 out]
              }
              frame False {
              }
            }
          }
          frame "Maximize", "Maximized" {
            w293 = T1."Maximized" ("State")
            n116 = property class="VI"(reference=w299, error in=w298) -> (reference out=w296:refnum<vi>, error out=w297:errorcluster, "FP.State"=w295:T1)
            n117 = Not Equal?(x=w295, y=w293) -> (x != y?=w294:bool)
            n118 = case shown="True" w294 {
              tunnel: [w304 w305] -> w300
              tunnel: w297 -> [w303 w305]
              tunnel: w296 -> [w302 _]
              tunnel: w293 -> [w301 _]
              frame True {
                n119 = invoke class="VI" method="FP.Open"(reference=w302, error in=w303, "State"=w301) -> (error out=w304:errorcluster)  [unwired: 2 in, 4 out]
              }
              frame False {
              }
            }
          }
        }
        n120 = call <vilib>:"Add State(s) to Queue__jki_lib_state_machine.vi"("State(s) in (\"\")"=w240) -> ("States Out"=w239:string)  [unwired: 14 in]
      }
      frame "---------- Macro ----------" {
        # "Do not put any code in this frame.\n(It is a separator no-op. You can make a copy of this frame to create a new Macro frame)"
        n121 = call <vilib>:"Add State(s) to Queue__jki_lib_state_machine.vi"("State(s) in (\"\")"=w309) -> ("States Out"=w308:string)  [unwired: 14 in]
      }
      frame "Macro: Initialize" {
        # "Initialization Macro\n(This is called once, when the VI starts)"
        n122 = call <vilib>:"Add State(s) to Queue__jki_lib_state_machine.vi"("State(s) in Front (\"\")"="Data: Initialize\nInitialize Core Data\nUI: Initialize\nUI: Front Panel State >> Open\nData: Initialize Top Level\nData: Reset Index\n//Measure: Temperature\n//Measure: Magnet\n//Measure: Capacitance\nUI: Clear Graph\nSweep: Initialize\nMacro: Sweep", "State(s) in (\"\")"=w314) -> ("States Out"=w313:string)  [unwired: 13 in]
      }
      frame "Macro: Sweep" {
        # "stop if true"
        # "continue if true"
        # "sweep is finished"
        # "keep sweeping"
        # "Do not put any code in this frame.\n(It is a separator no-op. You can make a copy of this frame to create a new Macro frame)"
        n123 = Unbundle By Name(w329) -> ("size"=w330:i32, "index"=w333:i32)
        n124 = Decrement(x=w330) -> (x-1=w323:i32)
        n125 = local read "stop"() -> (w316:bool)
        n126 = Not Equal?(x=w323, y=w333) -> (x != y?=w318:bool)
        n127 = Not(x=w316) -> (.not. x?=w317:bool)
        n128 = And(x=w317, y=w318) -> (x .and. y?=w315:bool)
        n129 = Select(t="Data: Reset Index\nConfigure: Set" ("State(s) in Front (\"\")"), s="set \"Vsg\" to initial value?", f="" ("State(s) in Front (\"\")")) -> (s? t:f=w320:string)
        n130 = call <vilib>:"Add State(s) to Queue__jki_lib_state_machine.vi"("State(s) in Front (\"\")"="File: Save" ("State(s) in Front (\"\")"), "State(s) in (\"\")"=w320, "State(s) at Back (\"\")"="Macro: Exit" ("State(s) in Front (\"\")")) -> ("States Out"=w324:string)  [unwired: 12 in]
        n131 = Select(t="Macro: Sweep" ("State(s) in Front (\"\")"), s=w315, f=w324) -> (s? t:f=w332:string)
        n132 = call <vilib>:"Add State(s) to Queue__jki_lib_state_machine.vi"("State(s) in Front (\"\")"="Configure: Set\nConfigure: Wait\nMeasure: Lockin\nMeasure: Time\n//Measure: Temperature\nUI: Update Graphs\nUI: Update Timer\nData: Increment Index" ("State(s) in Front (\"\")"), "State(s) at Back (\"\")"=w332) -> ("States Out"=w322:string)  [unwired: 13 in]
        n133 = call <vilib>:"Add State(s) to Queue__jki_lib_state_machine.vi"("State(s) in (\"\")"=w336, "State(s) at Back (\"\")"=w322) -> ("States Out"=w335:string)  [unwired: 13 in]
      }
      frame "Macro: Exit" {
        # "Exit Macro\n(This is called once, when the VI exits)"
        n134 = Unbundle By Name(w343) -> ("Core.Close Panel on Exit?"=w342:bool)
        n135 = Select(t="UI: Front Panel State >> Close", s=w342, f="") -> (s? t:f=w339:string)
        n136 = call <vilib>:"Add State(s) to Queue__jki_lib_state_machine.vi"("State(s) in (\"\")"=w339, "State(s) at Back (\"\")"="Data: Cleanup\nExit") -> ("States Out"=w337:string)  [unwired: 13 in]
        n137 = call <vilib>:"Add State(s) to Queue__jki_lib_state_machine.vi"("State(s) in Front (\"\")"=w337, "State(s) in (\"\")"=w346) -> ("States Out"=w345:string)  [unwired: 13 in]
      }
      frame "---------- Sweep ----------" {
        # "Do not put any code in this frame.\n(It is a separator no-op. You can make a copy of this frame to create a new Macro frame)"
        n138 = call <vilib>:"Add State(s) to Queue__jki_lib_state_machine.vi"("State(s) in (\"\")"=w350) -> ("States Out"=w349:string)  [unwired: 14 in]
      }
      frame "Sweep: Initialize" {
        w351 = 0.125 ("x")
        # "Converting Position to Voltage\n1V = 8um\n1um = 0.125V"
        # "define sweep"
        # "Do not put any code in this frame.\n(It is a separator no-op. You can make a copy of this frame to create a new Macro frame)"
        n139 = Unbundle By Name(w366) -> ("C.E."=w365:refnum<class "Control Experiment.lvclass">)
        n140 = Multiply(x=w351, y="End (um)") -> (x*y=w354:dbl)
        n141 = Multiply(x="Start (um)", y=w351) -> (x*y=w353:dbl)
        n142 = Multiply(x=w351, y="Step (um)") -> (x*y=w352:dbl)
        n143 = call <userlib>:"Max_Min_conversion.vi"("Min"=w353, "Max"=w354) -> ("offset"=w371:dbl, "Amplitude"=w370:dbl)  [unwired: 8 in]
        n144 = local read "Sweep"() -> (w355:enum16{"Vsg", "Vbg", "Z-height", ""})
        n145 = local read "Input"() -> (w358:i32[])
        n146 = call <userlib>:"Ramp.vi"("phase"="phase", "function (ramp)"="function (ramp)", "cycles (1,2,...)"="cycles (1,2,...)", "step size"=w352, "offset"=w371, "amplitude"=w370) -> ("Waveform Graph"=w367:dbl[])  [unwired: 3 in, 2 out]
        n147 = Format Into String(error in=w363, w355) -> (resulting string=w361:string, error out=w362:errorcluster)  [unwired: 2 in]
        n148 = call <userlib>:"Write Dictionary Element.vi"("error in (no error)"=w362, "value"=w367, "key"=w361, "Control Experiment in"=w365) -> ("error out"=w357:errorcluster, "Control Experiment out"=w360:refnum<class "Control Experiment.lvclass">)  [unwired: 6 in]
        n149 = case shown="\"Vsg\", Default" w355 {
          tunnel: w360 -> [w380 w386]
          tunnel: [w380 w385] -> w359
          tunnel: w358 -> [_ w384]
          tunnel: w357 -> [w379 w382]
          tunnel: [w379 w381] -> w356
          frame "Vbg" {
          }
          frame "Vsg", Default {
            n150 = call <userlib>:"Write Dictionary Element.vi"("error in (no error)"=w382, "value"=w384, "key"="Sweep Channels", "Control Experiment in"=w386) -> ("error out"=w381:errorcluster, "Control Experiment out"=w385:refnum<class "Control Experiment.lvclass">)  [unwired: 6 in]
          }
        }
        n151 = Array Size(array=w367) -> (size(s)=w364:i32)
        n152 = Bundle By Name(cluster=w366, "Sweep Values"=w367, "size"=w364, "C.E."=w359) -> (w369:T5)
        n153 = call <vilib>:"Add State(s) to Queue__jki_lib_state_machine.vi"("State(s) in (\"\")"=w378) -> ("States Out"=w377:string)  [unwired: 14 in]
      }
      frame "---------- Configure ----------" {
        # "Do not put any code in this frame.\n(It is a separator no-op. You can make a copy of this frame to create a new Macro frame)"
        n154 = call <vilib>:"Add State(s) to Queue__jki_lib_state_machine.vi"("State(s) in (\"\")"=w390) -> ("States Out"=w389:string)  [unwired: 14 in]
      }
      frame "Configure: Wait" {
        # "Do not put any code in this frame.\n(It is a separator no-op. You can make a copy of this frame to create a new Macro frame)"
        n155 = Unbundle By Name(w393) -> ("index"=w392:i32)
        n156 = case shown="Default" w392 {
          tunnel: ["Initial wait (ms)" "wait after setting Control (ms)"] -> w391
          frame 0 {
          }
          frame Default {
          }
        }
        n157 = call <userlib>:"Wait (ms)__ogtk.vi"("error in (no error)"=w395, "milliseconds to wait"=w391) -> ("error out"=w394:errorcluster)  [unwired: 8 in, 1 out]
        n158 = call <vilib>:"Add State(s) to Queue__jki_lib_state_machine.vi"("State(s) in (\"\")"=w397) -> ("States Out"=w396:string)  [unwired: 14 in]
      }
      frame "Configure: Set" {
        # "Do not put any code in this frame.\n(It is a separator no-op. You can make a copy of this frame to create a new Macro frame)"
        n159 = Unbundle By Name(w401) -> ("Instruments.Lockin"=w409:refnum<class "Instrument.Lockin.lvclass">, "Sweep Values"=w408:dbl[], "index"=w407:i32)
        n160 = Index Array(array=w408, index=w407) -> (element=w403:dbl)
        n161 = case shown="\"Vsg\", Default" "Sweep" {
          tunnel: w409 -> [w415 w449 w462]
          tunnel: w404 -> [w420 w448 w456]
          tunnel: w403 -> [w417 w445 w461]
          tunnel: [w419 w446 w453] -> w405
          tunnel: [w413 w444 w462] -> w400
          frame "Vsg", Default {
            n162 = call <userlib>:"getAO.vi"("Instrument.Lockin in"=w415) -> ("AOconfig"=w418:T9)  [unwired: 8 in, 2 out]
            n163 = Decrement(x="Input") -> (x-1=w414:i32[])
            n164 = for {
              tunnel: w417 -> [w442]
              shift-right: [w438] -> w412
              shift-left: w418 -> [w440]
              tunnel: w414 -> [w439] mode=indexing
              n165 = Index Array(array=w440, index=w439) -> (element=w443:T10)
              n166 = Bundle By Name(cluster=w443, "Offset"=w442) -> (w441:T10)
              n167 = Replace Array Subset(array=w440, new element=w441, index=w439) -> (w438:T9)
            }
            n168 = disable-structure shown="Enabled" {
              disable-tunnel: w420 -> [w426 w434]
              disable-tunnel: [w425 w433] -> w419
              disable-tunnel: w417 -> [w424 _]
              disable-tunnel: "Input" -> [w423 _]
              disable-tunnel: w415 -> [w422 w436]
              disable-tunnel: [w421 w435] -> w413
              disable-tunnel: w412 -> [_ w437]
              frame Disabled {
                n169 = for {
                  tunnel: w423 -> [w428] mode=indexing
                  tunnel: w424 -> [w427]
                  tunnel: w426 -> [w431]
                  tunnel: [w430] -> w425
                  shift-right: [w429] -> w421
                  shift-left: w422 -> [w432]
                  n170 = call <userlib>:"setAO_DC.vi"("error in (no error)"=w431, "DC (V)"=w427, "AO Channel"=w428, "Instrument.Lockin in"=w432) -> ("error out"=w430:errorcluster, "Instrument.Lockin out"=w429:refnum<class "Instrument.Lockin.lvclass">)  [unwired: 6 in]
                }
              }
              frame Enabled {
                n171 = call <userlib>:"setAO.vi"("error in (no error)"=w434, "Channels: AO"=w437, "Instrument.Lockin in"=w436) -> ("error out"=w433:errorcluster, "Instrument.Lockin out"=w435:refnum<class "Instrument.Lockin.lvclass">)  [unwired: 7 in]
              }
            }
          }
          frame "Vbg" {
            n172 = call <userlib>:"setAUX.vi"("error in (no error)"=w448, "AUX (V)"=w445, "Channel"=1, "Instrument.Lockin in"=w449) -> ("error out"=w446:errorcluster, "Instrument.Lockin out"=w444:refnum<class "Instrument.Lockin.lvclass">)  [unwired: 6 in]
          }
          frame "Z-height" {
            n173 = Number To Fractional String(number=w461, precision (6)=i16 7) -> (F-format string=w458:string)  [unwired: 2 in]
            n174 = call <userlib>:"Igor_OpenRefnum.vi"("error in (no error)"=w456) -> ("error out"=w450:errorcluster, "Application out"=w455:refnum<k7>)  [unwired: 9 in]
            n175 = Format Into String(format string="%s)" ("string"), initial string="td_WriteValue(\"A%Output\"," ("string"), w458) -> (resulting string=w454:string)  [unwired: 1 in, 1 out]
            n176 = call <userlib>:"Igor_SendCommand.vi"("error in (no error)"=w450, "command"=w454, "Application In"=w455) -> ("error out"=w451:errorcluster, "Application Out"=w452:refnum<k7>)  [unwired: 5 in, 2 out]
            n177 = call <userlib>:"Igor_CloseRefnum.vi"("error in (no error)"=w451, "Application"=w452) -> ("error out"=w453:errorcluster)  [unwired: 9 in]
          }
        }
        n178 = Bundle By Name(cluster=w401, "Instruments.Lockin"=w400) -> (w402:T5)
        n179 = call <vilib>:"Add State(s) to Queue__jki_lib_state_machine.vi"("State(s) in (\"\")"=w411) -> ("States Out"=w410:string)  [unwired: 14 in]
      }
      frame "---------- Measure ----------" {
        # "Template Separator\n(You can make a copy of, or modify, this frame)"
        n180 = call <vilib>:"Add State(s) to Queue__jki_lib_state_machine.vi"("State(s) in (\"\")"=w466) -> ("States Out"=w465:string)  [unwired: 14 in]
      }
      frame "Measure: Temperature" {
        # "Your code here.\n(You can make a copy of, or modify, this frame)"
        n181 = Unbundle By Name(w475) -> ("C.E."=w470:refnum<class "Control Experiment.lvclass">, "Instruments.Temperature"=w477:refnum<class "Instrument.Cryostat.lvclass">)
        n182 = call-dynamic "Get Temperature.vi"("error in (no error)"=w476, "Instrument.Cryostat in"=w477) -> ("error out"=w472:errorcluster, "Temperature (K)"=w468:dbl, "Instrument.Cryostat out"=w467:refnum<class "Instrument.Cryostat.lvclass">)  [unwired: 5 in, 2 out]
        "T (mK)" <- w468
        n183 = call <userlib>:"Write Dictionary Element.vi"("error in (no error)"=w472, "value"=w468, "key"="Temperature", "Control Experiment in"=w470) -> ("error out"=w471:errorcluster, "Control Experiment out"=w469:refnum<class "Control Experiment.lvclass">)  [unwired: 6 in]
        n184 = Bundle By Name(cluster=w475, "Instruments.Temperature"=w467, "C.E."=w469) -> (w474:T5)
        n185 = call <vilib>:"Add State(s) to Queue__jki_lib_state_machine.vi"("State(s) in (\"\")"=w479) -> ("States Out"=w478:string)  [unwired: 14 in]
      }
      frame "Measure: Magnet" {
        # "Your code here.\n(You can make a copy of, or modify, this frame)"
        n186 = Unbundle By Name(w489) -> ("C.E."=w485:refnum<class "Control Experiment.lvclass">, "Instruments.Magnet"=w490:refnum<class "Instrument.Cryostat.lvclass">)
        n187 = call-dynamic "Get Magnet.vi"("error in (no error)"=w487, "Instrument.Cryostat in"=w490) -> ("error out"=w482:errorcluster, "B Field (T)"=w484:dbl, "Instrument.Cryostat out"=w481:refnum<class "Instrument.Cryostat.lvclass">)  [unwired: 5 in, 2 out]
        "Field (T)" <- w484
        n188 = call <userlib>:"Write Dictionary Element.vi"("error in (no error)"=w482, "value"=w484, "key"="Magnet", "Control Experiment in"=w485) -> ("error out"=w483:errorcluster, "Control Experiment out"=w486:refnum<class "Control Experiment.lvclass">)  [unwired: 6 in]
        n189 = Bundle By Name(cluster=w489, "Instruments.Magnet"=w481, "C.E."=w486) -> (w488:T5)
        n190 = call <vilib>:"Add State(s) to Queue__jki_lib_state_machine.vi"("State(s) in (\"\")"=w492) -> ("States Out"=w491:string)  [unwired: 14 in]
      }
      frame "Measure: Capacitance" {
        # "Your code here.\n(You can make a copy of, or modify, this frame)"
        n191 = Unbundle By Name(w500) -> ("C.E."=w501:refnum<class "Control Experiment.lvclass">, "Instruments.Capacitance Bridge"=w503:refnum<class "Instrument.CBridge.lvclass">)
        n192 = call-dynamic "Get Capacitance.vi"("error in (no error)"=w497, "Instrument.CBridge in"=w503) -> ("error out"=w502:errorcluster, "Capacitance (pF)"=w493:dbl, "Instrument.CBridge out"=w494:refnum<class "Instrument.CBridge.lvclass">)  [unwired: 7 in]
        n193 = call <userlib>:"Write Dictionary Element.vi"("error in (no error)"=w502, "value"=w493, "key"="Capacitance", "Control Experiment in"=w501) -> ("error out"=w496:errorcluster, "Control Experiment out"=w498:refnum<class "Control Experiment.lvclass">)  [unwired: 6 in]
        n194 = Bundle By Name(cluster=w500, "Instruments.Capacitance Bridge"=w494, "C.E."=w498) -> (w499:T5)
        n195 = call <vilib>:"Add State(s) to Queue__jki_lib_state_machine.vi"("State(s) in (\"\")"=w505) -> ("States Out"=w504:string)  [unwired: 14 in]
      }
      frame "Measure: Lockin_old" {
        # "Template Separator\n(You can make a copy of, or modify, this frame)"
        n196 = Unbundle By Name(w518) -> ("C.E."=w517:refnum<class "Control Experiment.lvclass">, "Instruments.Lockin"=w520:refnum<class "Instrument.Lockin.lvclass">)
        n197 = call <userlib>:"waitForNewResults.vi"("error in (no error)"=w521, "Instrument.Lockin in"=w520) -> ("error out"=w515:errorcluster, "Results (Dictionary)"=w509:cluster{"key":string, "value":dbl}[], "Instrument.Lockin out"=w513:refnum<class "Instrument.Lockin.lvclass">)  [unwired: 7 in]
        n198 = call <userlib>:"Parse Results (all).vi"("Type"=Results_Type--Enum."Y", "Results (Dictionary)"=w509) -> ("Data"=w507:dbl[])  [unwired: 6 in, 3 out]
        n199 = call <userlib>:"Parse Results (all).vi"("Type"=Results_Type--Enum."Mean", "Results (Dictionary)"=w509) -> ("Data"=w506:dbl[])  [unwired: 6 in, 3 out]
        n200 = call <userlib>:"Parse Results (all).vi"("Type"=Results_Type--Enum."X", "Results (Dictionary)"=w509) -> ("Data"=w511:dbl[])  [unwired: 6 in, 3 out]
        n201 = for {
          tunnel: w511 -> [w539] mode=indexing
          tunnel: w507 -> [w534] mode=indexing
          tunnel: w515 -> [w533]
          tunnel: [w530] -> w514
          shift-right: [w531] -> w516
          shift-left: w517 -> [w542]
          tunnel: w506 -> [w526] mode=indexing
          i -> [w545]
          n202 = Increment(x=w545) -> (x+1=w529:i32)
          n203 = Format Into String(format string="X%d" ("wavenames"), error in=w533, w529) -> (resulting string=w541:string, error out=w537:errorcluster)  [unwired: 1 in]
          n204 = call <userlib>:"Append Dictionary Element.vi"("error in (no error)"=w537, "value"=w539, "key"=w541, "Control Experiment in"=w542) -> ("error out"=w536:errorcluster, "Control Experiment out"=w538:refnum<class "Control Experiment.lvclass">)  [unwired: 6 in]
          n205 = Format Into String(format string="Y%d" ("wavenames"), error in=w536, w529) -> (resulting string=w540:string, error out=w535:errorcluster)  [unwired: 1 in]
          n206 = call <userlib>:"Append Dictionary Element.vi"("error in (no error)"=w535, "value"=w534, "key"=w540, "Control Experiment in"=w538) -> ("error out"=w525:errorcluster, "Control Experiment out"=w532:refnum<class "Control Experiment.lvclass">)  [unwired: 6 in]
          n207 = Format Into String(format string="Mean%d" ("wavenames"), error in=w525, w529) -> (resulting string=w527:string, error out=w524:errorcluster)  [unwired: 1 in]
          n208 = call <userlib>:"Append Dictionary Element.vi"("error in (no error)"=w524, "value"=w526, "key"=w527, "Control Experiment in"=w532) -> ("error out"=w530:errorcluster, "Control Experiment out"=w531:refnum<class "Control Experiment.lvclass">)  [unwired: 6 in]
        }
        n209 = Bundle By Name(cluster=w518, "Instruments.Lockin"=w513, "Results (Dictionary)"=w509, "C.E."=w516) -> (w519:T5)
        n210 = call <vilib>:"Add State(s) to Queue__jki_lib_state_machine.vi"("State(s) in (\"\")"=w523) -> ("States Out"=w522:string)  [unwired: 14 in]
      }
      frame "Measure: Lockin" {
        # "Template Separator\n(You can make a copy of, or modify, this frame)"
        n211 = Unbundle By Name(w552) -> ("C.E."=w549:refnum<class "Control Experiment.lvclass">, "Instruments.Lockin"=w551:refnum<class "Instrument.Lockin.lvclass">)
        n212 = call <userlib>:"getResults.vi"("error in (no error)"=w547, "Instrument.Lockin in"=w551) -> ("error out"=w546:errorcluster, "Results (Dictionary)"=w550:cluster{"key":string, "value":dbl}[], "Instrument.Lockin out"=w548:refnum<class "Instrument.Lockin.lvclass">)  [unwired: 6 in, 1 out]
        n213 = Bundle By Name(cluster=w552, "Instruments.Lockin"=w548, "Results (Dictionary)"=w550, "C.E."=w549) -> (w553:T5)
        n214 = call <vilib>:"Add State(s) to Queue__jki_lib_state_machine.vi"("State(s) in (\"\")"=w555) -> ("States Out"=w554:string)  [unwired: 14 in]
      }
      frame "Measure: Time" {
        # "Your code here.\n(You can make a copy of, or modify, this frame)"
        n215 = Unbundle By Name(w562) -> ("C.E."=w561:refnum<class "Control Experiment.lvclass">)
        n216 = Get Date/Time In Seconds() -> (seconds since 1Jan1904=w564:timestamp)
        n217 = To Double Precision Float(number=w564) -> (double precision float=w559:dbl)
        n218 = call <userlib>:"Write Dictionary Element.vi"("error in (no error)"=w558, "value"=w559, "key"="Time", "Control Experiment in"=w561) -> ("error out"=w557:errorcluster, "Control Experiment out"=w560:refnum<class "Control Experiment.lvclass">)  [unwired: 6 in]
        n219 = Bundle By Name(cluster=w562, "C.E."=w560) -> (w563:T5)
        n220 = call <vilib>:"Add State(s) to Queue__jki_lib_state_machine.vi"("State(s) in (\"\")"=w566) -> ("States Out"=w565:string)  [unwired: 14 in]
      }
      frame "---------- File ----------" {
        # "Template Separator\n(You can make a copy of, or modify, this frame)"
        n221 = call <vilib>:"Add State(s) to Queue__jki_lib_state_machine.vi"("State(s) in (\"\")"=w570) -> ("States Out"=w569:string)  [unwired: 14 in]
      }
      frame "File: Configure" {
        # "Template Separator\n(You can make a copy of, or modify, this frame)"
        n222 = call <vilib>:"Add State(s) to Queue__jki_lib_state_machine.vi"("State(s) in (\"\")"=w574) -> ("States Out"=w573:string)  [unwired: 14 in]
      }
      frame "File: Save" {
        # "Template Separator\n(You can make a copy of, or modify, this frame)"
        n223 = Unbundle By Name(w577) -> ("C.E."=w581:refnum<class "Control Experiment.lvclass">, "Execution:State"=w578:T6)
        n224 = call <userlib>:"Exec State to Append.vi"("Execution:State"=w578) -> ()  [unwired: 2 in, 1 out]
        n225 = call <userlib>:"Save Transport TDMS File.vi"("error in (no error)"=w579, "Control Experiment in"=w581) -> ("error out"=w580:errorcluster, "Control Experiment out"=w575:refnum<class "Control Experiment.lvclass">)  [unwired: 8 in]
        n226 = Bundle By Name(cluster=w577, "C.E."=w575) -> (w576:T5)
        n227 = call <vilib>:"Add State(s) to Queue__jki_lib_state_machine.vi"("State(s) in (\"\")"=w583) -> ("States Out"=w582:string)  [unwired: 14 in]
      }
    }
  }
  "error out" <- w2
  n228 = Unbundle By Name(w4) -> ("Transport"=→"Transport.lvclass":refnum<class "Transport.lvclass">)
